vi "Script Configuration.vi"   [LabVIEW 2017]
uses:
  Classes/Configuration Session/Configuration Session.lvclass
  Components/Transceivers/UDP/Configuration/UDP Thread Configuration.lvclass
  Components/Transceivers/UDP/Configuration/Thread Settings.ctl
  Typedefs/DSF Timing Info.ctl
  DSF Core.lvlib
  Typedefs/DSF Core Plugin Configuration.ctl
  Typedefs/DSF Version Info.ctl
  Typedefs/DSF Settings Info.ctl
  Typedefs/DSF Core Thread Configuration.ctl
  Typedefs/DSF Direction.ctl
  Typedefs/DSF Timeout Behavior.ctl
  Typedefs/DSF Core Group Configuration.ctl
  Typedefs/DSF Core Transfer Configuration.ctl
  Typedefs/DSF Data Type.ctl
  Typedefs/DSF Core Channel Configuration.ctl
  Typedefs/DSF Engine Channel Configuration.ctl
  Typedefs/DSF Engine Transfer Configuration.ctl
  Typedefs/DSF Engine Transfer Group Configuration.ctl
  Typedefs/DSF Engine Plugin Thread Configuration.ctl
  Typedefs/DSF Engine Plugin Configuration.ctl
types:
  T1 = typedef "DSF Core.lvlib/DSF Engine Plugin Configuration.ctl" = cluster{"core":T2, "component settings":T4[], "threads":T6[]}
  T2 = typedef "DSF Core.lvlib/DSF Core Plugin Configuration.ctl" = cluster{"name":string, "components":string[], "cycle timing":T3}
  T3 = typedef "DSF Core.lvlib/DSF Timing Info.ctl" = cluster{"priority":u64, "decimation":u64, "offset":u64}
  T4 = typedef "DSF Core.lvlib/DSF Settings Info.ctl" = cluster{"component":string, "version":T5, "values":cluster{"key":string, "value":string}[]}
  T5 = typedef "DSF Core.lvlib/DSF Version Info.ctl" = cluster{"major":u32, "minor":u32, "fix":u32, "build":string}
  T6 = typedef "DSF Core.lvlib/DSF Engine Plugin Thread Configuration.ctl" = cluster{"core":T7, "component settings":T4[], "transfer groups":T8[]}
  T7 = typedef "DSF Core.lvlib/DSF Core Thread Configuration.ctl" = cluster{"processor":i32, "priority offset":i16}
  T8 = typedef "DSF Core.lvlib/DSF Engine Transfer Group Configuration.ctl" = cluster{"core":T9, "component settings":T4[], "transfers":T12[]}
  T9 = typedef "DSF Core.lvlib/DSF Core Group Configuration.ctl" = cluster{"name":string, "direction":T10, "cycle timing":T3, "timeout behavior":T11}
  T10 = typedef "DSF Core.lvlib/DSF Direction.ctl" = enum8{"Tx", "Rx"}
  T11 = typedef "DSF Core.lvlib/DSF Timeout Behavior.ctl" = enum8{"Increment Late Count", "Throw Error"}
  T12 = typedef "DSF Core.lvlib/DSF Engine Transfer Configuration.ctl" = cluster{"core":T13, "component settings":T4[], "channels":T14[]}
  T13 = typedef "DSF Core.lvlib/DSF Core Transfer Configuration.ctl" = cluster{"name":string}
  T14 = typedef "DSF Core.lvlib/DSF Engine Channel Configuration.ctl" = cluster{"core":T15, "component settings":T4[]}
  T15 = typedef "DSF Core.lvlib/DSF Core Channel Configuration.ctl" = cluster{"name":string, "units":string, "engine data type":T16, "string data type":T16, "string offset":u64}
  T16 = typedef "DSF Core.lvlib/DSF Data Type.ctl" = enum8{"Bool", "SGL", "DBL", "I8", "I16", "I32", "I64", "U8", "U16", "U32", "U64"}
  T17 = typedef "DSF Core.lvlib/UDP Thread Configuration.lvclass/Thread Settings.ctl" = cluster{"local port":u16, "local address":u32}
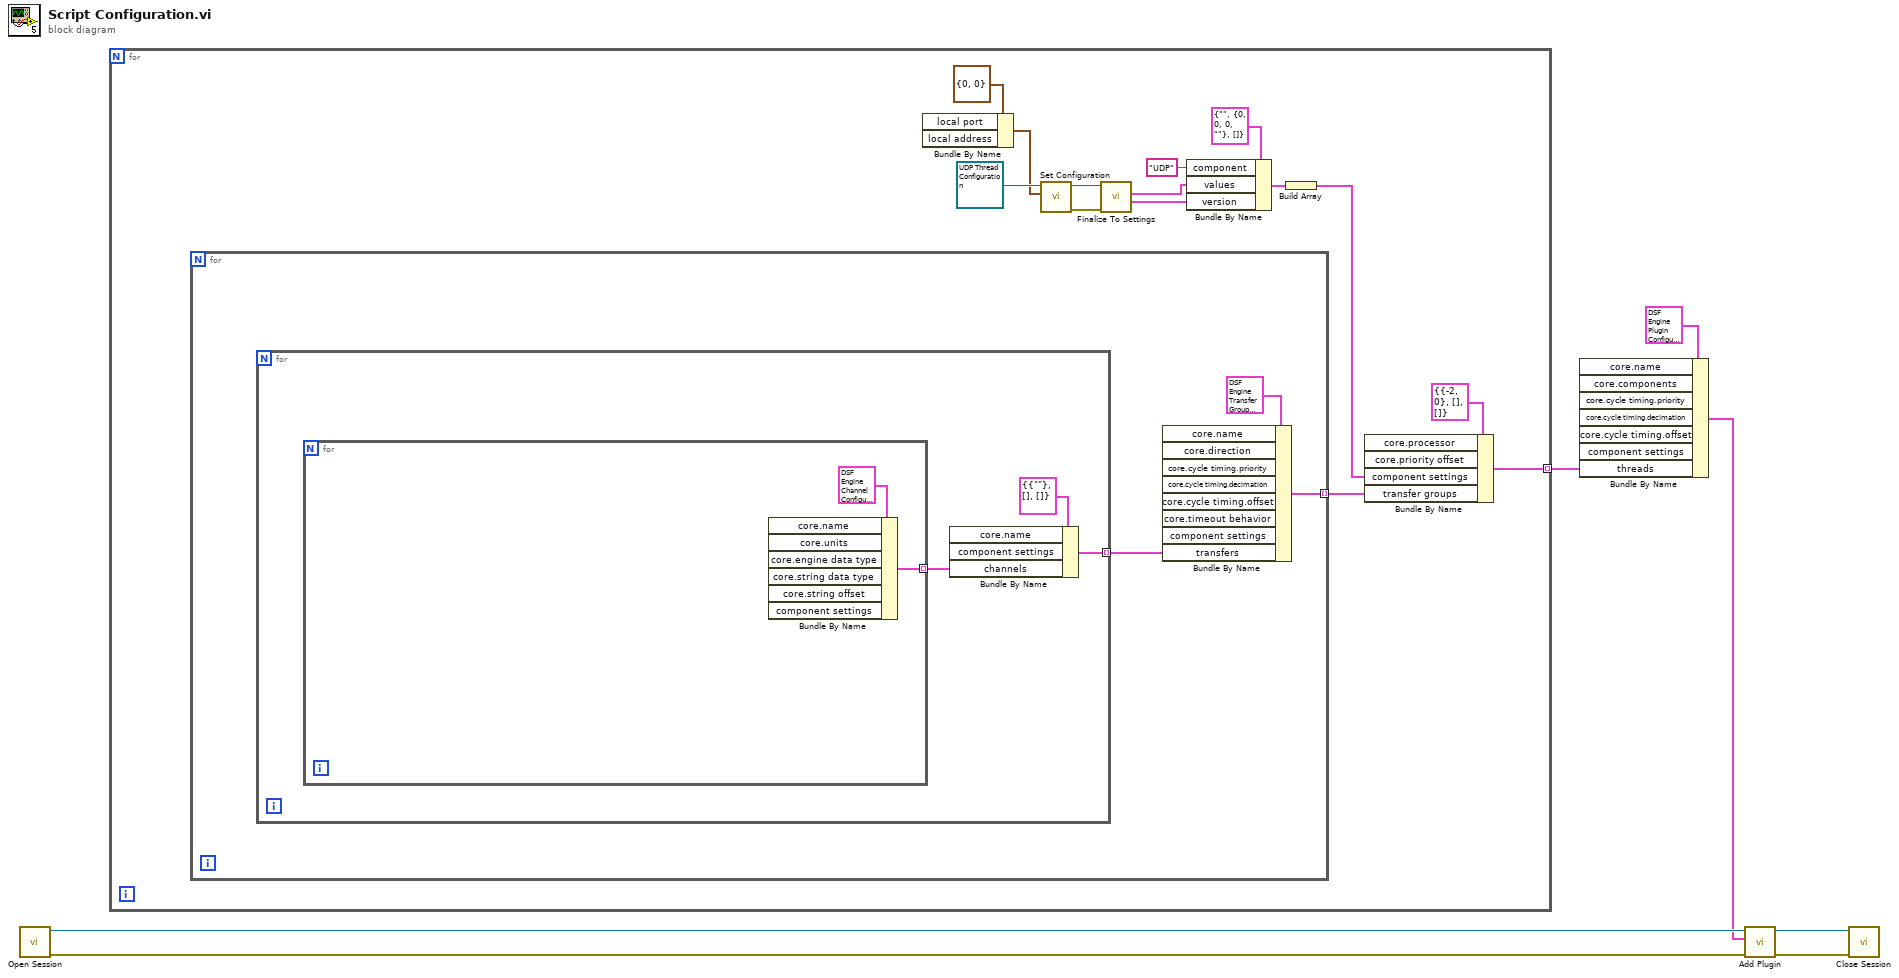
[diagram p0: block diagram]
diagram:
  n1 = call "Open Session.vi"() -> ("error out"=w5:errorcluster, "configuration session"=w7:refnum<class "Configuration Session.lvclass">)  [unwired: 7 in, 3 out]
  n2 = for {
    tunnel: [w20] -> w1 mode=indexing
    n3 = for {
      tunnel: [w23] -> w19 mode=indexing
      n4 = for {
        tunnel: [w26] -> w22 mode=indexing
        n5 = for {
          tunnel: [w28] -> w25 mode=indexing
          n6 = Bundle By Name(cluster=T14 {"core"={"name"="Channel", "units"="V", "engine data type"=enum."DBL", "string data type"=enum."DBL", "string offset"=0}, "component settings"=[]} ("channels")) -> (w28:T14)  [unwired: 6 in]
        }
        n7 = Bundle By Name(cluster=T12 {"core"={"name"=""}, "component settings"=[], "channels"=[]} ("Transfer Configuration"), "channels"=w25) -> (w26:T12)  [unwired: 2 in]
      }
      n8 = Bundle By Name(cluster=T8 {"core"={"name"="", "direction"=enum."Tx", "cycle timing"={"priority"=0, "decimation"=0, "offset"=0}, "timeout behavior"=enum."Increment Late Count"}, "component settings"=[], "transfers"=[]} ("Transfer Group Configuration"), "transfers"=w22) -> (w23:T8)  [unwired: 7 in]
    }
    n9 = Bundle By Name(cluster=T17 {"local port"=0, "local address"=0} ("thread settings")) -> (w13:T17)  [unwired: 2 in]
    n10 = call "Set Configuration.vi"("thread settings"=w13, "DSF UDP Thread Configuration in"=refnum<class "UDP Thread Configuration.lvclass"> refnum ("DSF Core.lvlib:DSF UDP Thread Configuration")) -> ("error out"=w17:errorcluster, "DSF UDP Thread Configuration out"=w18:refnum<class "UDP Thread Configuration.lvclass">)  [unwired: 8 in]
    n11 = call-dynamic "Finalize To Settings.vi"("error in (no error)"=w17, "UDP Thread Configuration in"=w18) -> ("settings version"=w11:T5, "settings"=w12:cluster{"key":string, "value":string}[])  [unwired: 6 in, 2 out]
    n12 = Bundle By Name(cluster=T4 {"component"="", "version"={"major"=0, "minor"=0, "fix"=0, "build"=""}, "values"=[]} ("component settings"), "component"="UDP", "values"=w12, "version"=w11) -> (w9:T4)
    n13 = Build Array(w9) -> (w8:T4[])
    n14 = Bundle By Name(cluster=T6 {"core"={"processor"=-2, "priority offset"=0}, "component settings"=[], "transfer groups"=[]} ("threads"), "component settings"=w8, "transfer groups"=w19) -> (w20:T6)  [unwired: 2 in]
  }
  n15 = Bundle By Name(cluster=T1 {"core"={"name"="Plugin", "components"=[], "cycle timing"={"priority"=10000, "decimation"=1, "offset"=0}}, "component settings"=[], "threads"=[]} ("plugin"), "threads"=w1) -> (w2:T1)  [unwired: 6 in]
  n16 = call "Add Plugin.vi"("error in (no error)"=w5, "plugin"=w2, "configuration session in"=w7) -> ("error out"=w4:errorcluster, "configuration session out"=w6:refnum<class "Configuration Session.lvclass">)  [unwired: 4 in, 2 out]
  n17 = call "Close Session.vi"("error in (no error)"=w4, "configuration session"=w6) -> ()  [unwired: 8 in, 2 out]
